vi "My Host.vi"() -> ()   [LabVIEW 2021]
panel:
  out "Button0":bool
  in  "stop":bool
  in  "Set FPGA LED":bool
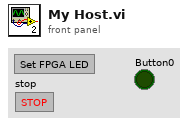
[diagram p1: front panel]
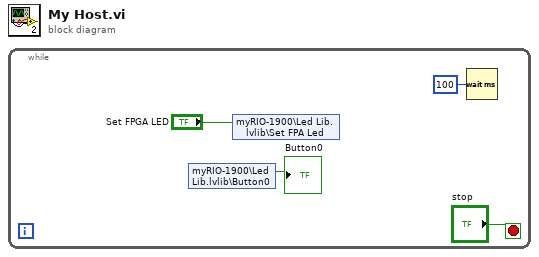
[diagram p0: block diagram]
diagram:
  n1 = while {
    stop <- "stop" stop-if-true
    n2 = shared-variable "myRIO-1900\\Led Lib.lvlib\\Button0"() -> (→"Button0":bool)  [unwired: 1 in, 1 out]
    n3 = shared-variable "myRIO-1900\\Led Lib.lvlib\\Set FPA Led"("Set FPGA LED") -> ()  [unwired: 1 in, 1 out]
    n4 = Wait (ms)(milliseconds to wait=u32 100) -> ()  [unwired: 1 out]
  }
